vi "Write PCM CAN ID.vi"(8 "error in (no error)":errorcluster, 10 "PCM CAN ID":u8, 11 "Comp Pressure in":refnum<class "Comp Pressure.lvclass">) -> (0 "error out":errorcluster, 3 "Comp Pressure out":refnum<class "Comp Pressure.lvclass">)   [LabVIEW 2014, in "Comp Pressure.lvlib" / "Comp Pressure.lvclass"]
uses:
  Comp Pressure.lvclass
  Comp Pressure.lvclass/Comp Pressure.ctl
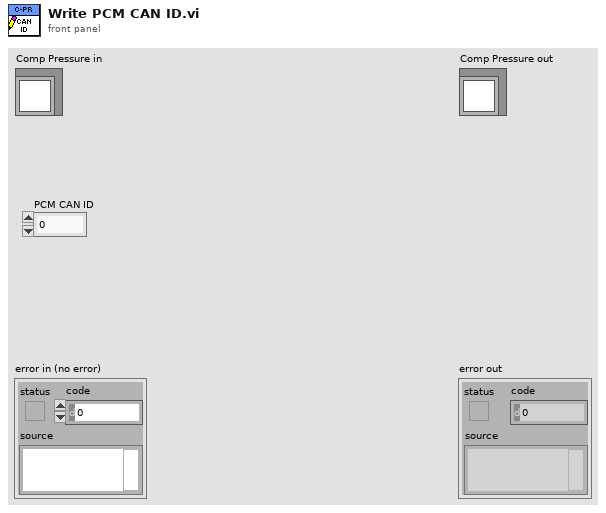
[diagram p1: front panel]
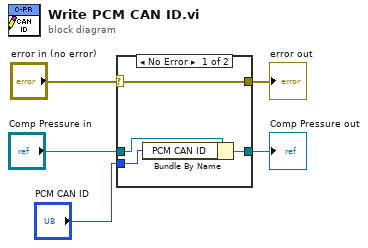
[diagram p0: block diagram]
diagram:
  n1 = case shown="No Error" "error in (no error)" {
    selector: "error in (no error)" -> [w9 w10]
    tunnel: [w9 w10] -> w4
    tunnel: [w7 w11] -> w2
    tunnel: "Comp Pressure in" -> [w8 w11]
    tunnel: "PCM CAN ID" -> [w6 _]
    frame No Error {
      n2 = Bundle By Name(cluster=w8, "PCM CAN ID"=w6) -> (w7:refnum<class "Comp Pressure.lvclass">)
    }
    frame Error {
    }
  }
  "error out" <- w4
  "Comp Pressure out" <- w2
